vi "DisplayJson.vi"(11 "JSON String In":string="[{\"version\":\"1.0.0\",\"header\":{\"creationDate\":\"2022-06-03T00:00:00\",\"remarks\":\"\",\"serialNumber\":\"98172\",\"productNumber\":\"123021.1804\",\"productType\":\"PAA-9L\",\"pressureType\":2,\"productSeries\":\"9L\",\"compensatedTemperatureRange\":{\"min\":-10.0,\"max\":80.0,\"unit\":4},\"compensatedPressureRange\":{\"min\":0.0,\"max\":0.35,\"unit\":3},\"electricSupply\":{\"magnitude\":1.0,\"unit\":18},\"orderNumber\":9990266,\"orderPosition\":3,\"orderTargetDispatchDate\":\"2022-06-02T00:00:00+00:00\",\"customerName\":\"DemoData Inc.\",\"customerNumber\":12345678,\"customerOrderNumber\":\"Cust-9990266-123\",\"customerReferenceNumber\":\"\",\"customerProductT...") -> ()   [LabVIEW 2017] (continued)
\"temperature\":{\"output\":{\"magnitude\":19.5449,\"unit\":4},\"error\":{\"magnitude\":-0.0059422599,\"unit\":4}}}}}},{\"reference\":\"F_12300_XX_0000098765\",\"environmentTarget\":{\"pressure\":{\"magnitude\":0.11,\"unit\":3},\"temperature\":{\"magnitude\":20.0,\"unit\":4}},\"environment\":{\"pressure\":{\"magnitude\":0.11,\"unit\":3},\"temperature\":{\"magnitude\":19.5509,\"unit\":4},\"supply\":{\"magnitude\":1.0,\"unit\":18}},\"raw\":{\"signal\":{\"magnitude\":26.416661534,\"unit\":22},\"bridgeResistance\":{\"magnitude\":3495.5999199,\"unit\":28}},\"compensated\":{\"mathematicalModels\":{\"MM0123\":{\"pressure\":{\"output\":{\"magnitude\":0.109977,\"unit\":3},\"error\":{\"magnitude\":-0.0065360975,\"unit\":7}},\"temperature\":{\"output\":{\"magnitude\":19.5426,\"unit\":4},\"error\":{\"magnitude\":-0.0082689775,\"unit\":4}}}}}},{\"reference\":\"F_12300_XX_0000098765\",\"environmentTarget\":{\"pressure\":{\"magnitude\":0.19,\"unit\":3},\"temperature\":{\"magnitude\":20.0,\"unit\":4}},\"environment\":{\"pressure\":{\"magnitude\":0.189998,\"unit\":3},\"temperature\":{\"magnitude\":19.5509,\"unit\":4},\"supply\":{\"magnitude\":1.0,\"unit\":18}},\"raw\":{\"signal\":{\"magnitude\":37.030268769,\"unit\":22},\"bridgeResistance\":{\"magnitude\":3491.6224563,\"unit\":28}},\"compensated\":{\"mathematicalModels\":{\"MM0123\":{\"pressure\":{\"output\":{\"magnitude\":0.190007,\"unit\":3},\"error\":{\"magnitude\":0.0024560994,\"unit\":7}},\"temperature\":{\"output\":{\"magnitude\":19.5389,\"unit\":4},\"error\":{\"magnitude\":-0.012049357,\"unit\":4}}}}}},{\"reference\":\"F_12300_XX_0000098765\",\"environmentTarget\":{\"pressure\":{\"magnitude\":0.27,\"unit\":3},\"temperature\":{\"magnitude\":20.0,\"unit\":4}},\"environment\":{\"pressure\":{\"magnitude\":0.269994,\"unit\":3},\"temperature\":{\"magnitude\":19.5509,\"unit\":4},\"supply\":{\"magnitude\":1.0,\"unit\":18}},\"raw\":{\"signal\":{\"magnitude\":47.60635601,\"unit\":22},\"bridgeResistance\":{\"magnitude\":3487.7228678,\"unit\":28}},\"compensated\":{\"mathematicalModels\":{\"MM0123\":{\"pressure\":{\"output\":{\"magnitude\":0.270015,\"unit\":3},\"error\":{\"magnitude\":0.0061300393,\"unit\":7}},\"temperature\":{\"output\":{\"magnitude\":19.5358,\"unit\":4},\"error\":{\"magnitude\":-0.015037284,\"unit\":4}}}}}},{\"reference\":\"F_12300_XX_0000098765\",\"environmentTarget\":{\"pressure\":{\"magnitude\":0.35,\"unit\":3},\"temperature\":{\"magnitude\":20.0,\"unit\":4}},\"environment\":{\"pressure\":{\"magnitude\":0.35,\"unit\":3},\"temperature\":{\"magnitude\":19.5509,\"unit\":4},\"supply\":{\"magnitude\":1.0,\"unit\":18}},\"raw\":{\"signal\":{\"magnitude\":58.14484892,\"unit\":22},\"bridgeResistance\":{\"magnitude\":3483.890155,\"unit\":28}},\"compensated\":{\"mathematicalModels\":{\"MM0123\":{\"pressure\":{\"output\":{\"magnitude\":0.350003,\"unit\":3},\"error\":{\"magnitude\":0.00098441802,\"unit\":7}},\"temperature\":{\"output\":{\"magnitude\":19.5323,\"unit\":4},\"error\":{\"magnitude\":-0.018584481,\"unit\":4}}}}}},{\"reference\":\"F_12300_XX_0000098765\",\"environmentTarget\":{\"pressure\":{\"magnitude\":0.03,\"unit\":3},\"temperature\":{\"magnitude\":40.0,\"unit\":4}},\"environment\":{\"pressure\":{\"magnitude\":0.0300037,\"unit\":3},\"temperature\":{\"magnitude\":39.7284,\"unit\":4},\"supply\":{\"magnitude\":1.0,\"unit\":18}},\"raw\":{\"signal\":{\"magnitude\":16.748092375,\"unit\":22},\"bridgeResistance\":{\"magnitude\":3674.5848343,\"unit\":28}},\"compensated\":{\"mathematicalModels\":{\"MM0123\":{\"pressure\":{\"output\":{\"magnitude\":0.0300189,\"unit\":3},\"error\":{\"magnitude\":0.004330657,\"unit\":7}},\"temperature\":{\"output\":{\"magnitude\":39.7229,\"unit\":4},\"error\":{\"magnitude\":-0.005475721,\"unit\":4}}}}}},{\"reference\":\"F_12300_XX_0000098765\",\"environmentTarget\":{\"pressure\":{\"magnitude\":0.11,\"unit\":3},\"temperature\":{\"magnitude\":40.0,\"unit\":4}},\"environment\":{\"pressure\":{\"magnitude\":0.110002,\"unit\":3},\"temperature\":{\"magnitude\":39.7284,\"unit\":4},\"supply\":{\"magnitude\":1.0,\"unit\":18}},\"raw\":{\"signal\":{\"magnitude\":27.434150149,\"unit\":22},\"bridgeResistance\":{\"magnitude\":3670.5212952,\"unit\":28}},\"compensated\":{\"mathematicalModels\":{\"MM0123\":{\"pressure\":{\"output\":{\"magnitude\":0.109982,\"unit\":3},\"error\":{\"magnitude\":-0.0057516302,\"unit\":7}},\"temperature\":{\"output\":{\"magnitude\":39.7229,\"unit\":4},\"error\":{\"magnitude\":-0.0055694235,\"unit\":4}}}}}},{\"reference\":\"F_12300_XX_0000098765\",\"environmentTarget\":{\"pressure\":{\"magnitude\":0.19,\"unit\":3},\"temperature\":{\"magnitude\":40.0,\"unit\":4}},\"environment\":{\"pressure\":{\"magnitude\":0.190005,\"unit\":3},\"temperature\":{\"magnitude\":39.7284,\"unit\":4},\"supply\":{\"magnitude\":1.0,\"unit\":18}},\"raw\":{\"signal\":{\"magnitude\":38.097016772,\"unit\":22},\"bridgeResistance\":{\"magnitude\":3666.4814116,\"unit\":28}},\"compensated\":{\"mathematicalModels\":{\"MM0123\":{\"pressure\":{\"output\":{\"magnitude\":0.190006,\"unit\":3},\"error\":{\"magnitude\":0.0004046361,\"unit\":7}},\"temperature\":{\"output\":{\"magnitude\":39.7178,\"unit\":4},\"error\":{\"magnitude\":-0.010669287,\"unit\":4}}}}}},{\"reference\":\"F_12300_XX_0000098765\",\"environmentTarget\":{\"pressure\":{\"magnitude\":0.27,\"unit\":3},\"temperature\":{\"magnitude\":40.0,\"unit\":4}},\"environment\":{\"pressure\":{\"magnitude\":0.269997,\"unit\":3},\"temperature\":{\"magnitude\":39.7284,\"unit\":4},\"supply\":{\"magnitude\":1.0,\"unit\":18}},\"raw\":{\"signal\":{\"magnitude\":48.726177501,\"unit\":22},\"bridgeResistance\":{\"magnitude\":3662.5874392,\"unit\":28}},\"compensated\":{\"mathematicalModels\":{\"MM0123\":{\"pressure\":{\"output\":{\"magnitude\":0.270008,\"unit\":3},\"error\":{\"magnitude\":0.0031543513,\"unit\":7}},\"temperature\":{\"output\":{\"magnitude\":39.7206,\"unit\":4},\"error\":{\"magnitude\":-0.0078327671,\"unit\":4}}}}}},{\"reference\":\"F_12300_XX_0000098765\",\"environmentTarget\":{\"pressure\":{\"magnitude\":0.35,\"unit\":3},\"temperature\":{\"magnitude\":40.0,\"unit\":4}},\"environment\":{\"pressure\":{\"magnitude\":0.350003,\"unit\":3},\"temperature\":{\"magnitude\":39.7284,\"unit\":4},\"supply\":{\"magnitude\":1.0,\"unit\":18}},\"raw\":{\"signal\":{\"magnitude\":59.320792825,\"unit\":22},\"bridgeResistance\":{\"magnitude\":3658.7134123,\"unit\":28}},\"compensated\":{\"mathematicalModels\":{\"MM0123\":{\"pressure\":{\"output\":{\"magnitude\":0.349986,\"unit\":3},\"error\":{\"magnitude\":-0.0048622518,\"unit\":7}},\"temperature\":{\"output\":{\"magnitude\":39.7176,\"unit\":4},\"error\":{\"magnitude\":-0.010854606,\"unit\":4}}}}}},{\"reference\":\"F_12300_XX_0000098765\",\"environmentTarget\":{\"pressure\":{\"magnitude\":0.03,\"unit\":3},\"temperature\":{\"magnitude\":60.0,\"unit\":4}},\"environment\":{\"pressure\":{\"magnitude\":0.0299911,\"unit\":3},\"temperature\":{\"magnitude\":59.8651,\"unit\":4},\"supply\":{\"magnitude\":1.0,\"unit\":18}},\"raw\":{\"signal\":{\"magnitude\":17.813294413,\"unit\":22},\"bridgeResistance\":{\"magnitude\":3866.6561439,\"unit\":28}},\"compensated\":{\"mathematicalModels\":{\"MM0123\":{\"pressure\":{\"output\":{\"magnitude\":0.0299973,\"unit\":3},\"error\":{\"magnitude\":0.0017700015,\"unit\":7}},\"temperature\":{\"output\":{\"magnitude\":59.9259,\"unit\":4},\"error\":{\"magnitude\":0.06081023,\"unit\":4}}}}}},{\"reference\":\"F_12300_XX_0000098765\",\"environmentTarget\":{\"pressure\":{\"magnitude\":0.11,\"unit\":3},\"temperature\":{\"magnitude\":60.0,\"unit\":4}},\"environment\":{\"pressure\":{\"magnitude\":0.109995,\"unit\":3},\"temperature\":{\"magnitude\":59.8651,\"unit\":4},\"supply\":{\"magnitude\":1.0,\"unit\":18}},\"raw\":{\"signal\":{\"magnitude\":28.584875218,\"unit\":22},\"bridgeResistance\":{\"magnitude\":3862.5400232,\"unit\":28}},\"compensated\":{\"mathematicalModels\":{\"MM0123\":{\"pressure\":{\"output\":{\"magnitude\":0.109979,\"unit\":3},\"error\":{\"magnitude\":-0.0046951087,\"unit\":7}},\"temperature\":{\"output\":{\"magnitude\":59.9272,\"unit\":4},\"error\":{\"magnitude\":0.062078048,\"unit\":4}}}}}},{\"reference\":\"F_12300_XX_0000098765\",\"environmentTarget\":{\"pressure\":{\"magnitude\":0.19,\"unit\":3},\"temperature\":{\"magnitude\":60.0,\"unit\":4}},\"environment\":{\"pressure\":{\"magnitude\":0.190004,\"unit\":3},\"temperature\":{\"magnitude\":59.8651,\"unit\":4},\"supply\":{\"magnitude\":1.0,\"unit\":18}},\"raw\":{\"signal\":{\"magnitude\":39.33493725,\"unit\":22},\"bridgeResistance\":{\"magnitude\":3858.4848982,\"unit\":28}},\"compensated\":{\"mathematicalModels\":{\"MM0123\":{\"pressure\":{\"output\":{\"magnitude\":0.190003,\"unit\":3},\"error\":{\"magnitude\":-0.00025005669,\"unit\":7}},\"temperature\":{\"output\":{\"magnitude\":59.9287,\"unit\":4},\"error\":{\"magnitude\":0.063577803,\"unit\":4}}}}}},{\"reference\":\"F_12300_XX_0000098765\",\"environmentTarget\":{\"pressure\":{\"magnitude\":0.27,\"unit\":3},\"temperature\":{\"magnitude\":60.0,\"unit\":4}},\"environment\":{\"pressure\":{\"magnitude\":0.270004,\"unit\":3},\"temperature\":{\"magnitude\":59.8651,\"unit\":4},\"supply\":{\"magnitude\":1.0,\"unit\":18}},\"raw\":{\"signal\":{\"magnitude\":50.057189453,\"unit\":22},\"bridgeResistance\":{\"magnitude\":3854.4965821,\"unit\":28}},\"compensated\":{\"mathematicalModels\":{\"MM0123\":{\"pressure\":{\"output\":{\"magnitude\":0.270024,\"unit\":3},\"error\":{\"magnitude\":0.0057789716,\"unit\":7}},\"temperature\":{\"output\":{\"magnitude\":59.9307,\"unit\":4},\"error\":{\"magnitude\":0.065552658,\"unit\":4}}}}}},{\"reference\":\"F_12300_XX_0000098765\",\"environmentTarget\":{\"pressure\":{\"magnitude\":0.35,\"unit\":3},\"temperature\":{\"magnitude\":60.0,\"unit\":4}},\"environment\":{\"pressure\":{\"magnitude\":0.349995,\"unit\":3},\"temperature\":{\"magnitude\":59.8651,\"unit\":4},\"supply\":{\"magnitude\":1.0,\"unit\":18}},\"raw\":{\"signal\":{\"magnitude\":60.744545032,\"unit\":22},\"bridgeResistance\":{\"magnitude\":3850.5667489,\"unit\":28}},\"compensated\":{\"mathematicalModels\":{\"MM0123\":{\"pressure\":{\"output\":{\"magnitude\":0.349989,\"unit\":3},\"error\":{\"magnitude\":-0.0016070127,\"unit\":7}},\"temperature\":{\"output\":{\"magnitude\":59.9319,\"unit\":4},\"error\":{\"magnitude\":0.06679753,\"unit\":4}}}}}},{\"reference\":\"F_12300_XX_0000098765\",\"environmentTarget\":{\"pressure\":{\"magnitude\":0.03,\"unit\":3},\"temperature\":{\"magnitude\":80.0,\"unit\":4}},\"environment\":{\"pressure\":{\"magnitude\":0.0300046,\"unit\":3},\"temperature\":{\"magnitude\":79.9513,\"unit\":4},\"supply\":{\"magnitude\":1.0,\"unit\":18}},\"raw\":{\"signal\":{\"magnitude\":19.002144905,\"unit\":22},\"bridgeResistance\":{\"magnitude\":4072.8231737,\"unit\":28}},\"compensated\":{\"mathematicalModels\":{\"MM0123\":{\"pressure\":{\"output\":{\"magnitude\":0.0300206,\"unit\":3},\"error\":{\"magnitude\":0.004584639,\"unit\":7}},\"temperature\":{\"output\":{\"magnitude\":80.0436,\"unit\":4},\"error\":{\"magnitude\":0.092214141,\"unit\":4}}}}}},{\"reference\":\"F_12300_XX_0000098765\",\"environmentTarget\":{\"pressure\":{\"magnitude\":0.11,\"unit\":3},\"temperature\":{\"magnitude\":80.0,\"unit\":4}},\"environment\":{\"pressure\":{\"magnitude\":0.110002,\"unit\":3},\"temperature\":{\"magnitude\":79.9513,\"unit\":4},\"supply\":{\"magnitude\":1.0,\"unit\":18}},\"raw\":{\"signal\":{\"magnitude\":29.879764386,\"unit\":22},\"bridgeResistance\":{\"magnitude\":4068.6482783,\"unit\":28}},\"compensated\":{\"mathematicalModels\":{\"MM0123\":{\"pressure\":{\"output\":{\"magnitude\":0.109968,\"unit\":3},\"error\":{\"magnitude\":-0.0096781592,\"unit\":7}},\"temperature\":{\"output\":{\"magnitude\":80.0462,\"unit\":4},\"error\":{\"magnitude\":0.094857113,\"unit\":4}}}}}},{\"reference\":\"F_12300_XX_0000098765\",\"environmentTarget\":{\"pressure\":{\"magnitude\":0.19,\"unit\":3},\"temperature\":{\"magnitude\":80.0,\"unit\":4}},\"environment\":{\"pressure\":{\"magnitude\":0.189994,\"unit\":3},\"temperature\":{\"magnitude\":79.9513,\"unit\":4},\"supply\":{\"magnitude\":1.0,\"unit\":18}},\"raw\":{\"signal\":{\"magnitude\":40.746012852,\"unit\":22},\"bridgeResistance\":{\"magnitude\":4064.5654978,\"unit\":28}},\"compensated\":{\"mathematicalModels\":{\"MM0123\":{\"pressure\":{\"output\":{\"magnitude\":0.190002,\"unit\":3},\"error\":{\"magnitude\":0.0022412163,\"unit\":7}},\"temperature\":{\"output\":{\"magnitude\":80.0536,\"unit\":4},\"error\":{\"magnitude\":0.1022268,\"unit\":4}}}}}},{\"reference\":\"F_12300_XX_0000098765\",\"environmentTarget\":{\"pressure\":{\"magnitude\":0.27,\"unit\":3},\"temperature\":{\"magnitude\":80.0,\"unit\":4}},\"environment\":{\"pressure\":{\"magnitude\":0.270005,\"unit\":3},\"temperature\":{\"magnitude\":79.9513,\"unit\":4},\"supply\":{\"magnitude\":1.0,\"unit\":18}},\"raw\":{\"signal\":{\"magnitude\":51.587537274,\"unit\":22},\"bridgeResistance\":{\"magnitude\":4060.5136813,\"unit\":28}},\"compensated\":{\"mathematicalModels\":{\"MM0123\":{\"pressure\":{\"output\":{\"magnitude\":0.270027,\"unit\":3},\"error\":{\"magnitude\":0.0064070438,\"unit\":7}},\"temperature\":{\"output\":{\"magnitude\":80.0595,\"unit\":4},\"error\":{\"magnitude\":0.10820001,\"unit\":4}}}}}},{\"reference\":\"F_12300_XX_0000098765\",\"environmentTarget\":{\"pressure\":{\"magnitude\":0.35,\"unit\":3},\"temperature\":{\"magnitude\":80.0,\"unit\":4}},\"environment\":{\"pressure\":{\"magnitude\":0.349997,\"unit\":3},\"temperature\":{\"magnitude\":79.9513,\"unit\":4},\"supply\":{\"magnitude\":1.0,\"unit\":18}},\"raw\":{\"signal\":{\"magnitude\":62.396098066,\"unit\":22},\"bridgeResistance\":{\"magnitude\":4056.4915818,\"unit\":28}},\"compensated\":{\"mathematicalModels\":{\"MM0123\":{\"pressure\":{\"output\":{\"magnitude\":0.349985,\"unit\":3},\"error\":{\"magnitude\":-0.0034619433,\"unit\":7}},\"temperature\":{\"output\":{\"magnitude\":80.0638,\"unit\":4},\"error\":{\"magnitude\":0.11240626,\"unit\":4}}}}}}]},{\"version\":\"1.0.0\",\"header\":{\"creationDate\":\"2022-06-03T00:00:00\",\"remarks\":\"\",\"serialNumber\":\"98083\",\"productNumber\":\"123021.1804\",\"productType\":\"PAA-9L\",\"pressureType\":2,\"productSeries\":\"9L\",\"compensatedTemperatureRange\":{\"min\":-10.0,\"max\":80.0,\"unit\":4},\"compensatedPressureRange\":{\"min\":0.0,\"max\":0.35,\"unit\":3},\"electricSupply\":{\"magnitude\":1.0,\"unit\":18},\"orderNumber\":9990266,\"orderPosition\":3,\"orderTargetDispatchDate\":\"2022-06-02T00:00:00+00:00\",\"customerName\":\"DemoData Inc.\",\"customerNumber\":12345678,\"customerOrderNumber\":\"Cust-9990266-123\",\"customerReferenceNumber\":\"\",\"customerProductType\":\"123021-1804 Rev.AA\"},\"compensationMethods\":{\"mathematicalModels\":{\"MM0123\":{\"modelType\":\"MM0123\",\"productNumber\":\"000000.0000\",\"compensatedTemperatureRange\":{\"min\":-10.0,\"max\":80.0,\"unit\":4},\"compensatedPressureRange\":{\"min\":0.0,\"max\":0.35,\"unit\":3},\"electricSupply\":{\"magnitude\":1.0,\"unit\":18},\"parts\":{\"pressure\":{\"inputs\":[\"Sig\",\"R\"],\"output\":\"P\",\"description\":\"P = f(Sig,R)\",\"coefficients\":[[3.63310435718,-0.00363389206026,1.34930392587E-06,-2.24563835828E-10,1.39905821744E-14],[-0.0993877484134,0.000105975761375,-3.95803321041E-08,6.56139178036E-12,-4.08510736386E-16],[-0.000366248546746,4.19017408478E-07,-1.77205627573E-10,3.30128020446E-14,-2.29210272903E-18]]},\"temperature\":{\"inputs\":[\"R\",\"Sig\"],\"output\":\"T\",\"description\":\"T = f(R,Sig)\",\"coefficients\":[[-7824.08516559,-7.6450274546,0.0655428608171],[7.6820085907,0.00943972080923,-7.29339544197E-05],[-0.0028951031634,-4.23164182833E-06,3.02382272713E-08],[4.94544252506E-07,8.27138238584E-10,-5.54321442715E-12],[-3.18956234296E-11,-5.97910707007E-14,3.79410156991E-16]]}}}}},\"measurements\":[{\"reference\":\"F_12300_XX_0000098765\",\"environmentTarget\":{\"pressure\":{\"magnitude\":0.03,\"unit\":3},\"temperature\":{\"magnitude\":-10.0,\"unit\":4}},\"environment\":{\"pressure\":{\"magnitude\":0.029998,\"unit\":3},\"temperature\":{\"magnitude\":-10.7286,\"unit\":4},\"supply\":{\"magnitude\":1.0,\"unit\":18}},\"raw\":{\"signal\":{\"magnitude\":15.768740367,\"unit\":22},\"bridgeResistance\":{\"magnitude\":3289.7518235,\"unit\":28}},\"compensated\":{\"mathematicalModels\":{\"MM0123\":{\"pressure\":{\"output\":{\"magnitude\":0.0300118,\"unit\":3},\"error\":{\"magnitude\":0.0039552178,\"unit\":7}},\"temperature\":{\"output\":{\"magnitude\":-10.8423,\"unit\":4},\"error\":{\"magnitude\":-0.11370704,\"unit\":4}}}}}},{\"reference\":\"F_12300_XX_0000098765\",\"environmentTarget\":{\"pressure\":{\"magnitude\":0.11,\"unit\":3},\"temperature\":{\"magnitude\":-10.0,\"unit\":4}},\"environment\":{\"pressure\":{\"magnitude\":0.110009,\"unit\":3},\"temperature\":{\"magnitude\":-10.7286,\"unit\":4},\"supply\":{\"magnitude\":1.0,\"unit\":18}},\"raw\":{\"signal\":{\"magnitude\":27.663432001,\"unit\":22},\"bridgeResistance\":{\"magnitude\":3284.2425899,\"unit\":28}},\"compensated\":{\"mathematicalModels\":{\"MM0123\":{\"pressure\":{\"output\":{\"magnitude\":0.109973,\"unit\":3},\"error\":{\"magnitude\":-0.010313162,\"unit\":7}},\"temperature\":{\"output\":{\"magnitude\":-10.8468,\"unit\":4},\"error\":{\"magnitude\":-0.1181895,\"unit\":4}}}}}},{\"reference\":\"F_12300_XX_0000098765\",\"environmentTarget\":{\"pressure\":{\"magnitude\":0.19,\"unit\":3},\"temperature\":{\"magnitude\":-10.0,\"unit\":4}},\"environment\":{\"pressure\":{\"magnitude\":0.190006,\"unit\":3},\"temperature\":{\"magnitude\":-10.7286,\"unit\":4},\"supply\":{\"magnitude\":1.0,\"unit\":18}},\"raw\":{\"signal\":{\"magnitude\":39.521415848,\"unit\":22},\"bridgeResistance\":{\"magnitude\":3279.8976313,\"unit\":28}},\"compensated\":{\"mathematicalModels\":{\"MM0123\":{\"pressure\":{\"output\":{\"magnitude\":0.190016,\"unit\":3},\"error\":{\"magnitude\":0.0029939943,\"unit\":7}},\"temperature\":{\"output\":{\"magnitude\":-10.8438,\"unit\":4},\"error\":{\"magnitude\":-0.11516709,\"unit\":4}}}}}},{\"reference\":\"F_12300_XX_0000098765\",\"environmentTarget\":{\"pressure\":{\"magnitude\":0.27,\"unit\":3},\"temperature\":{\"magnitude\":-10.0,\"unit\":4}},\"environment\":{\"pressure\":{\"magnitude\":0.270006,\"unit\":3},\"temperature\":{\"magnitude\":-10.7286,\"unit\":4},\"supply\":{\"magnitude\":1.0,\"unit\":18}},\"raw\":{\"signal\":{\"magnitude\":51.326682167,\"unit\":22},\"bridgeResistance\":{\"magnitude\":3275.6600996,\"unit\":28}},\"compensated\":{\"mathematicalModels\":{\"MM0123\":{\"pressure\":{\"output\":{\"magnitude\":0.270037,\"unit\":3},\"error\":{\"magnitude\":0.0089972975,\"unit\":7}},\"temperature\":{\"output\":{\"magnitude\":-10.8382,\"unit\":4},\"error\":{\"magnitude\":-0.10956906,\"unit\":4}}}}}},{\"reference\":\"F_12300_XX_0000098765\",\"environmentTarget\":{\"pressure\":{\"magnitude\":0.35,\"unit\":3},\"temperature\":{\"magnitude\":-10.0,\"unit\":4}},\"environment\":{\"pressure\":{\"magnitude\":0.35,\"unit\":3},\"temperature\":{\"magnitude\":-10.7286,\"unit\":4},\"supply\":{\"magnitude\":1.0,\"unit\":18}},\"raw\":{\"signal\":{\"magnitude\":63.072780161,\"unit\":22},\"bridgeResistance\":{\"magnitude\":3271.4490528,\"unit\":28}},\"compensated\":{\"mathematicalModels\":{\"MM0123\":{\"pressure\":{\"output\":{\"magnitude\":0.349995,\"unit\":3},\"error\":{\"magnitude\":-0.0014930458,\"unit\":7}},\"temperature\":{\"output\":{\"magnitude\":-10.8469,\"unit\":4},\"error\":{\"magnitude\":-0.11824585,\"unit\":4}}}}}},{\"reference\":\"F_12300_XX_0000098765\",\"environmentTarget\":{\"pressure\":{\"magnitude\":0.03,\"unit\":3},\"temperature\":{\"magnitude\":0.0,\"unit\":4}},\"environment\":{\"pressure\":{\"magnitude\":0.0299993,\"unit\":3},\"temperature\":{\"magnitude\":-0.629962,\"unit\":4},\"supply\":{\"magnitude\":1.0,\"unit\":18}},\"raw\":{\"signal\":{\"magnitude\":16.265941035,\"unit\":22},\"bridgeResistance\":{\"magnitude\":3359.1605663,\"unit\":28}},\"compensated\":{\"mathematicalModels\":{\"MM0123\":{\"pressure\":{\"output\":{\"magnitude\":0.0300172,\"unit\":3},\"error\":{\"magnitude\":0.0051262489,\"unit\":7}},\"temperature\":{\"output\":{\"magnitude\":-0.751572,\"unit\":4},\"error\":{\"magnitude\":-0.1216099,\"unit\":4}}}}}},{\"reference\":\"F_12300_XX_0000098765\",\"environmentTarget\":{\"pressure\":{\"magnitude\":0.11,\"unit\":3},\"temperature\":{\"magnitude\":0.0,\"unit\":4}},\"environment\":{\"pressure\":{\"magnitude\":0.110001,\"unit\":3},\"temperature\":{\"magnitude\":-0.629962,\"unit\":4},\"supply\":{\"magnitude\":1.0,\"unit\":18}},\"raw\":{\"signal\":{\"magnitude\":28.125684179,\"unit\":22},\"bridgeResistance\":{\"magnitude\":3354.6447949,\"unit\":28}},\"compensated\":{\"mathematicalModels\":{\"MM0123\":{\"pressure\":{\"output\":{\"magnitude\":0.109972,\"unit\":3},\"error\":{\"magnitude\":-0.0083468924,\"unit\":7}},\"temperature\":{\"output\":{\"magnitude\":-0.756891,\"unit\":4},\"error\":{\"magnitude\":-0.12692921,\"unit\":4}}}}}},{\"reference\":\"F_12300_XX_0000098765\",\"environmentTarget\":{\"pressure\":{\"magnitude\":0.19,\"unit\":3},\"temperature\":{\"magnitude\":0.0,\"unit\":4}},\"environment\":{\"pressure\":{\"magnitude\":0.190006,\"unit\":3},\"temperature\":{\"magnitude\":-0.629962,\"unit\":4},\"supply\":{\"magnitude\":1.0,\"unit\":18}},\"raw\":{\"signal\":{\"magnitude\":39.949259633,\"unit\":22},\"bridgeResistance\":{\"magnitude\":3350.2650804,\"unit\":28}},\"compensated\":{\"mathematicalModels\":{\"MM0123\":{\"pressure\":{\"output\":{\"magnitude\":0.19,\"unit\":3},\"error\":{\"magnitude\":-0.001845037,\"unit\":7}},\"temperature\":{\"output\":{\"magnitude\":-0.757234,\"unit\":4},\"error\":{\"magnitude\":-0.12727247,\"unit\":4}}}}}},{\"reference\":\"F_12300_XX_0000098765\",\"environmentTarget\":{\"pressure\":{\"magnitude\":0.27,\"unit\":3},\"temperature\":{\"magnitude\":0.0,\"unit\":4}},\"environment\":{\"pressure\":{\"magnitude\":0.269995,\"unit\":3},\"temperature\":{\"magnitude\":-0.629962,\"unit\":4},\"supply\":{\"magnitude\":1.0,\"unit\":18}},\"raw\":{\"signal\":{\"magnitude\":51.72348672,\"unit\":22},\"bridgeResistance\":{\"magnitude\":3345.9485402,\"unit\":28}},\"compensated\":{\"mathematicalModels\":{\"MM0123\":{\"pressure\":{\"output\":{\"magnitude\":0.270016,\"unit\":3},\"error\":{\"magnitude\":0.0058723742,\"unit\":7}},\"temperature\":{\"output\":{\"magnitude\":-0.763469,\"unit\":4},\"error\":{\"magnitude\":-0.1335069,\"unit\":4}}}}}},{\"reference\":\"F_12300_XX_0000098765\",\"environmentTarget\":{\"pressure\":{\"magnitude\":0.35,\"unit\":3},\"temperature\":{\"magnitude\":0.0,\"unit\":4}},\"environment\":{\"pressure\":{\"magnitude\":0.350003,\"unit\":3},\"temperature\":{\"magnitude\":-0.629962,\"unit\":4},\"supply\":{\"magnitude\":1.0,\"unit\":18}},\"raw\":{\"signal\":{\"magnitude\":63.441446846,\"unit\":22},\"bridgeResistance\":{\"magnitude\":3341.7747282,\"unit\":28}},\"compensated\":{\"mathematicalModels\":{\"MM0123\":{\"pressure\":{\"output\":{\"magnitude\":0.34997,\"unit\":3},\"error\":{\"magnitude\":-0.009570085,\"unit\":7}},\"temperature\":{\"output\":{\"magnitude\":-0.765087,\"unit\":4},\"error\":{\"magnitude\":-0.1351251,\"unit\":4}}}}}},{\"reference\":\"F_12300_XX_0000098765\",\"environmentTarget\":{\"pressure\":{\"magnitude\":0.03,\"unit\":3},\"temperature\":{\"magnitude\":20.0,\"unit\":4}},\"environment\":{\"pressure\":{\"magnitude\":0.0299954,\"unit\":3},\"temperature\":{\"magnitude\":19.5509,\"unit\":4},\"supply\":{\"magnitude\":1.0,\"unit\":18}},\"raw\":{\"signal\":{\"magnitude\":17.297816417,\"unit\":22},\"bridgeResistance\":{\"magnitude\":3516.9951878,\"unit\":28}},\"compensated\":{\"mathematicalModels\":{\"MM0123\":{\"pressure\":{\"output\":{\"magnitude\":0.0300062,\"unit\":3},\"error\":{\"magnitude\":0.0030915574,\"unit\":7}},\"temperature\":{\"output\":{\"magnitude\":19.5472,\"unit\":4},\"error\":{\"magnitude\":-0.0036683152,\"unit\":4}}}}}},{\"reference\":\"F_12300_XX_0000098765\",\"environmentTarget\":{\"pressure\":{\"magnitude\":0.11,\"unit\":3},\"temperature\":{\"magnitude\":20.0,\"unit\":4}},\"environment\":{\"pressure\":{\"magnitude\":0.109995,\"unit\":3},\"temperature\":{\"magnitude\":19.5509,\"unit\":4},\"supply\":{\"magnitude\":1.0,\"unit\":18}},\"raw\":{\"signal\":{\"magnitude\":29.147457751,\"unit\":22},\"bridgeResistance\":{\"magnitude\":3512.4984667,\"unit\":28}},\"compensated\":{\"mathematicalModels\":{\"MM0123\":{\"pressure\":{\"output\":{\"magnitude\":0.109965,\"unit\":3},\"error\":{\"magnitude\":-0.0084408516,\"unit\":7}},\"temperature\":{\"output\":{\"magnitude\":19.543,\"unit\":4},\"error\":{\"magnitude\":-0.0078639068,\"unit\":4}}}}}},{\"reference\":\"F_12300_XX_0000098765\",\"environmentTarget\":{\"pressure\":{\"magnitude\":0.19,\"unit\":3},\"temperature\":{\"magnitude\":20.0,\"unit\":4}},\"environment\":{\"pressure\":{\"magnitude\":0.190002,\"unit\":3},\"temperature\":{\"magnitude\":19.5509,\"unit\":4},\"supply\":{\"magnitude\":1.0,\"unit\":18}},\"raw\":{\"signal\":{\"magnitude\":40.967596289,\"unit\":22},\"bridgeResistance\":{\"magnitude\":3508.1412376,\"unit\":28}},\"compensated\":{\"mathematicalModels\":{\"MM0123\":{\"pressure\":{\"output\":{\"magnitude\":0.190009,\"unit\":3},\"error\":{\"magnitude\":0.0019583559,\"unit\":7}},\"temperature\":{\"output\":{\"magnitude\":19.5457,\"unit\":4},\"error\":{\"magnitude\":-0.0051906945,\"unit\":4}}}}}},{\"reference\":\"F_12300_XX_0000098765\",\"environmentTarget\":{\"pressure\":{\"magnitude\":0.27,\"unit\":3},\"temperature\":{\"magnitude\":20.0,\"unit\":4}},\"environment\":{\"pressure\":{\"magnitude\":0.26999,\"unit\":3},\"temperature\":{\"magnitude\":19.5509,\"unit\":4},\"supply\":{\"magnitude\":1.0,\"unit\":18}},\"raw\":{\"signal\":{\"magnitude\":52.741361922,\"unit\":22},\"bridgeResistance\":{\"magnitude\":3503.7893624,\"unit\":28}},\"compensated\":{\"mathematicalModels\":{\"MM0123\":{\"pressure\":{\"output\":{\"magnitude\":0.270029,\"unit\":3},\"error\":{\"magnitude\":0.011218428,\"unit\":7}},\"temperature\":{\"output\":{\"magnitude\":19.538,\"unit\":4},\"error\":{\"magnitude\":-0.012843363,\"unit\":4}}}}}},{\"reference\":\"F_12300_XX_0000098765\",\"environmentTarget\":{\"pressure\":{\"magnitude\":0.35,\"unit\":3},\"temperature\":{\"magnitude\":20.0,\"unit\":4}},\"environment\":{\"pressure\":{\"magnitude\":0.350004,\"unit\":3},\"temperature\":{\"magnitude\":19.5509,\"unit\":4},\"supply\":{\"magnitude\":1.0,\"unit\":18}},\"raw\":{\"signal\":{\"magnitude\":64.467097155,\"unit\":22},\"bridgeResistance\":{\"magnitude\":3499.5857801,\"unit\":28}},\"compensated\":{\"mathematicalModels\":{\"MM0123\":{\"pressure\":{\"output\":{\"magnitude\":0.350009,\"unit\":3},\"error\":{\"magnitude\":0.0013639933,\"unit\":7}},\"temperature\":{\"output\":{\"magnitude\":19.5374,\"unit\":4},\"error\":{\"magnitude\":-0.013502905,\"unit\":4}}}}}},{\"reference\":\"F_12300_XX_0000098765\",\"environmentTarget\":{\"pressure\":{\"magnitude\":0.03,\"unit\":3},\"temperature\":{\"magnitude\":40.0,\"unit\":4}},\"environment\":{\"pressure\":{\"magnitude\":0.0299955,\"unit\":3},\"temperature\":{\"magnitude\":39.7284,\"unit\":4},\"supply\":{\"magnitude\":1.0,\"unit\":18}},\"raw\":{\"signal\":{\"magnitude\":18.397808565,\"unit\":22},\"bridgeResistance\":{\"magnitude\":3693.5579638,\"unit\":28}},\"compensated\":{\"mathematicalModels\":{\"MM0123\":{\"pressure\":{\"output\":{\"magnitude\":0.0300132,\"unit\":3},\"error\":{\"magnitude\":0.0050623537,\"unit\":7}},\"temperature\":{\"output\":{\"magnitude\":39.7198,\"unit\":4},\"error\":{\"magnitude\":-0.0086558786,\"unit\":4}}}}}},{\"reference\":\"F_12300_XX_0000098765\",\"environmentTarget\":{\"pressure\":{\"magnitude\":0.11,\"unit\":3},\"temperature\":{\"magnitude\":40.0,\"unit\":4}},\"environment\":{\"pressure\":{\"magnitude\":0.109995,\"unit\":3},\"temperature\":{\"magnitude\":39.7284,\"unit\":4},\"supply\":{\"magnitude\":1.0,\"unit\":18}},\"raw\":{\"signal\":{\"magnitude\":30.299736541,\"unit\":22},\"bridgeResistance\":{\"magnitude\":3689.0769444,\"unit\":28}},\"compensated\":{\"mathematicalModels\":{\"MM0123\":{\"pressure\":{\"output\":{\"magnitude\":0.109963,\"unit\":3},\"error\":{\"magnitude\":-0.0091372216,\"unit\":7}},\"temperature\":{\"output\":{\"magnitude\":39.7197,\"unit\":4},\"error\":{\"magnitude\":-0.0087145955,\"unit\":4}}}}}},{\"reference\":\"F_12300_XX_0000098765\",\"environmentTarget\":{\"pressure\":{\"magnitude\":0.19,\"unit\":3},\"temperature\":{\"magnitude\":40.0,\"unit\":4}},\"environment\":{\"pressure\":{\"magnitude\":0.190004,\"unit\":3},\"temperature\":{\"magnitude\":39.7284,\"unit\":4},\"supply\":{\"magnitude\":1.0,\"unit\":18}},\"raw\":{\"signal\":{\"magnitude\":42.177555685,\"unit\":22},\"bridgeResistance\":{\"magnitude\":3684.6154146,\"unit\":28}},\"compensated\":{\"mathematicalModels\":{\"MM0123\":{\"pressure\":{\"output\":{\"magnitude\":0.190004,\"unit\":3},\"error\":{\"magnitude\":2.3318189E-05,\"unit\":7}},\"temperature\":{\"output\":{\"magnitude\":39.7145,\"unit\":4},\"error\":{\"magnitude\":-0.013875982,\"unit\":4}}}}}},{\"reference\":\"F_12300_XX_0000098765\",\"environmentTarget\":{\"pressure\":{\"magnitude\":0.27,\"unit\":3},\"temperature\":{\"magnitude\":40.0,\"unit\":4}},\"environment\":{\"pressure\":{\"magnitude\":0.269998,\"unit\":3},\"temperature\":{\"magnitude\":39.7284,\"unit\":4},\"supply\":{\"magnitude\":1.0,\"unit\":18}},\"raw\":{\"signal\":{\"magnitude\":54.013879922,\"unit\":22},\"bridgeResistance\":{\"magnitude\":3680.2587913,\"unit\":28}},\"compensated\":{\"mathematicalModels\":{\"MM0123\":{\"pressure\":{\"output\":{\"magnitude\":0.270016,\"unit\":3},\"error\":{\"magnitude\":0.0051611949,\"unit\":7}},\"temperature\":{\"output\":{\"magnitude\":39.7128,\"unit\":4},\"error\":{\"magnitude\":-0.015632767,\"unit\":4}}}}}},{\"reference\":\"F_12300_XX_0000098765\",\"environmentTarget\":{\"pressure\":{\"magnitude\":0.35,\"unit\":3},\"temperature\":{\"magnitude\":40.0,\"unit\":4}},\"environment\":{\"pressure\":{\"magnitude\":0.350002,\"unit\":3},\"temperature\":{\"magnitude\":39.7284,\"unit\":4},\"supply\":{\"magnitude\":1.0,\"unit\":18}},\"raw\":{\"signal\":{\"magnitude\":65.805074007,\"unit\":22},\"bridgeResistance\":{\"magnitude\":3675.994032,\"unit\":28}},\"compensated\":{\"mathematicalModels\":{\"MM0123\":{\"pressure\":{\"output\":{\"magnitude\":0.349974,\"unit\":3},\"error\":{\"magnitude\":-0.0078616514,\"unit\":7}},\"temperature\":{\"output\":{\"magnitude\":39.7128,\"unit\":4},\"error\":{\"magnitude\":-0.01561436,\"unit\":4}}}}}},{\"reference\":\"F_12300_XX_0000098765\",\"environmentTarget\":{\"pressure\":{\"magnitude\":0.03,\"unit\":3},\"temperature\":{\"magnitude\":60.0,\"unit\":4}},\"environment\":{\"pressure\":{\"magnitude\":0.0299999,\"unit\":3},\"temperature\":{\"magnitude\":59.8651,\"unit\":4},\"supply\":{\"magnitude\":1.0,\"unit\":18}},\"raw\":{\"signal\":{\"magnitude\":19.604034653,\"unit\":22},\"bridgeResistance\":{\"magnitude\":3896.2995143,\"unit\":28}},\"compensated\":{\"mathematicalModels\":{\"MM0123\":{\"pressure\":{\"output\":{\"magnitude\":0.0300139,\"unit\":3},\"error\":{\"magnitude\":0.0040132125,\"unit\":7}},\"temperature\":{\"output\":{\"magnitude\":59.9337,\"unit\":4},\"error\":{\"magnitude\":0.068596457,\"unit\":4}}}}}},{\"reference\":\"F_12300_XX_0000098765\",\"environmentTarget\":{\"pressure\":{\"magnitude\":0.11,\"unit\":3},\"temperature\":{\"magnitude\":60.0,\"unit\":4}},\"environment\":{\"pressure\":{\"magnitude\":0.109995,\"unit\":3},\"temperature\":{\"magnitude\":59.8651,\"unit\":4},\"supply\":{\"magnitude\":1.0,\"unit\":18}},\"raw\":{\"signal\":{\"magnitude\":31.600949028,\"unit\":22},\"bridgeResistance\":{\"magnitude\":3891.7514685,\"unit\":28}},\"compensated\":{\"mathematicalModels\":{\"MM0123\":{\"pressure\":{\"output\":{\"magnitude\":0.109965,\"unit\":3},\"error\":{\"magnitude\":-0.008619277,\"unit\":7}},\"temperature\":{\"output\":{\"magnitude\":59.9365,\"unit\":4},\"error\":{\"magnitude\":0.071398734,\"unit\":4}}}}}},{\"reference\":\"F_12300_XX_0000098765\",\"environmentTarget\":{\"pressure\":{\"magnitude\":0.19,\"unit\":3},\"temperature\":{\"magnitude\":60.0,\"unit\":4}},\"environment\":{\"pressure\":{\"magnitude\":0.190009,\"unit\":3},\"temperature\":{\"magnitude\":59.8651,\"unit\":4},\"supply\":{\"magnitude\":1.0,\"unit\":18}},\"raw\":{\"signal\":{\"magnitude\":43.579762231,\"unit\":22},\"bridgeResistance\":{\"magnitude\":3877.2639948,\"unit\":28}},\"compensated\":{\"mathematicalModels\":{\"MM0123\":{\"pressure\":{\"output\":{\"magnitude\":0.190016,\"unit\":3},\"error\":{\"magnitude\":0.0019454055,\"unit\":7}},\"temperature\":{\"output\":{\"magnitude\":59.9394,\"unit\":4},\"error\":{\"magnitude\":0.074263125,\"unit\":4}}}}}},{\"reference\":\"F_12300_XX_0000098765\",\"environmentTarget\":{\"pressure\":{\"magnitude\":0.27,\"unit\":3},\"temperature\":{\"magnitude\":60.0,\"unit\":4}},\"environment\":{\"pressure\":{\"magnitude\":0.270006,\"unit\":3},\"temperature\":{\"magnitude\":59.8651,\"unit\":4},\"supply\":{\"magnitude\":1.0,\"unit\":18}},\"raw\":{\"signal\":{\"magnitude\":55.520057917,\"unit\":22},\"bridgeResistance\":{\"magnitude\":3872.8109489,\"unit\":28}},\"compensated\":{\"mathematicalModels\":{\"MM0123\":{\"pressure\":{\"output\":{\"magnitude\":0.270032,\"unit\":3},\"error\":{\"magnitude\":0.0075675436,\"unit\":7}},\"temperature\":{\"output\":{\"magnitude\":59.9389,\"unit\":4},\"error\":{\"magnitude\":0.073763296,\"unit\":4}}}}}},{\"reference\":\"F_12300_XX_0000098765\",\"environmentTarget\":{\"pressure\":{\"magnitude\":0.35,\"unit\":3},\"temperature\":{\"magnitude\":60.0,\"unit\":4}},\"environment\":{\"pressure\":{\"magnitude\":0.349994,\"unit\":3},\"temperature\":{\"magnitude\":59.8651,\"unit\":4},\"supply\":{\"magnitude\":1.0,\"unit\":18}},\"raw\":{\"signal\":{\"magnitude\":67.418352287,\"unit\":22},\"bridgeResistance\":{\"magnitude\":3868.4767722,\"unit\":28}},\"compensated\":{\"mathematicalModels\":{\"MM0123\":{\"pressure\":{\"output\":{\"magnitude\":0.349987,\"unit\":3},\"error\":{\"magnitude\":-0.0021229316,\"unit\":7}},\"temperature\":{\"output\":{\"magnitude\":59.9434,\"unit\":4},\"error\":{\"magnitude\":0.078304539,\"unit\":4}}}}}},{\"reference\":\"F_12300_XX_0000098765\",\"environmentTarget\":{\"pressure\":{\"magnitude\":0.03,\"unit\":3},\"temperature\":{\"magnitude\":80.0,\"unit\":4}},\"environment\":{\"pressure\":{\"magnitude\":0.0299987,\"unit\":3},\"temperature\":{\"magnitude\":79.9513,\"unit\":4},\"supply\":{\"magnitude\":1.0,\"unit\":18}},\"raw\":{\"signal\":{\"magnitude\":20.96693822,\"unit\":22},\"bridgeResistance\":{\"magnitude\":4094.2798686,\"unit\":28}},\"compensated\":{\"mathematicalModels\":{\"MM0123\":{\"pressure\":{\"output\":{\"magnitude\":0.0300202,\"unit\":3},\"error\":{\"magnitude\":0.0061545516,\"unit\":7}},\"temperature\":{\"output\":{\"magnitude\":80.0538,\"unit\":4},\"error\":{\"magnitude\":0.10242499,\"unit\":4}}}}}},{\"reference\":\"F_12300_XX_0000098765\",\"environmentTarget\":{\"pressure\":{\"magnitude\":0.11,\"unit\":3},\"temperature\":{\"magnitude\":80.0,\"unit\":4}},\"environment\":{\"pressure\":{\"magnitude\":0.110013,\"unit\":3},\"temperature\":{\"magnitude\":79.9513,\"unit\":4},\"supply\":{\"magnitude\":1.0,\"unit\":18}},\"raw\":{\"signal\":{\"magnitude\":33.086392769,\"unit\":22},\"bridgeResistance\":{\"magnitude\":4089.6557362,\"unit\":28}},\"compensated\":{\"mathematicalModels\":{\"MM0123\":{\"pressure\":{\"output\":{\"magnitude\":0.109965,\"unit\":3},\"error\":{\"magnitude\":-0.013726951,\"unit\":7}},\"temperature\":{\"output\":{\"magnitude\":80.0564,\"unit\":4},\"error\":{\"magnitude\":0.10502604,\"unit\":4}}}}}},{\"reference\":\"F_12300_XX_0000098765\",\"environmentTarget\":{\"pressure\":{\"magnitude\":0.19,\"unit\":3},\"temperature\":{\"magnitude\":80.0,\"unit\":4}},\"environment\":{\"pressure\":{\"magnitude\":0.190002,\"unit\":3},\"temperature\":{\"magnitude\":79.9513,\"unit\":4},\"supply\":{\"magnitude\":1.0,\"unit\":18}},\"raw\":{\"signal\":{\"magnitude\":45.192919898,\"unit\":22},\"bridgeResistance\":{\"magnitude\":4085.123909,\"unit\":28}},\"compensated\":{\"mathematicalModels\":{\"MM0123\":{\"pressure\":{\"output\":{\"magnitude\":0.190006,\"unit\":3},\"error\":{\"magnitude\":0.0010687773,\"unit\":7}},\"temperature\":{\"output\":{\"magnitude\":80.0643,\"unit\":4},\"error\":{\"magnitude\":0.11293662,\"unit\":4}}}}}},{\"reference\":\"F_12300_XX_0000098765\",\"environmentTarget\":{\"pressure\":{\"magnitude\":0.27,\"unit\":3},\"temperature\":{\"magnitude\":80.0,\"unit\":4}},\"environment\":{\"pressure\":{\"magnitude\":0.270003,\"unit\":3},\"temperature\":{\"magnitude\":79.9513,\"unit\":4},\"supply\":{\"magnitude\":1.0,\"unit\":18}},\"raw\":{\"signal\":{\"magnitude\":57.271028109,\"unit\":22},\"bridgeResistance\":{\"magnitude\":4080.6383175,\"unit\":28}},\"compensated\":{\"mathematicalModels\":{\"MM0123\":{\"pressure\":{\"output\":{\"magnitude\":0.270045,\"unit\":3},\"error\":{\"magnitude\":0.011980425,\"unit\":7}},\"temperature\":{\"output\":{\"magnitude\":80.0724,\"unit\":4},\"error\":{\"magnitude\":0.12109066,\"unit\":4}}}}}},{\"reference\":\"F_12300_XX_0000098765\",\"environmentTarget\":{\"pressure\":{\"magnitude\":0.35,\"unit\":3},\"temperature\":{\"magnitude\":80.0,\"unit\":4}},\"environment\":{\"pressure\":{\"magnitude\":0.350001,\"unit\":3},\"temperature\":{\"magnitude\":79.9513,\"unit\":4},\"supply\":{\"magnitude\":1.0,\"unit\":18}},\"raw\":{\"signal\":{\"magnitude\":69.304666615,\"unit\":22},\"bridgeResistance\":{\"magnitude\":4076.1600415,\"unit\":28}},\"compensated\":{\"mathematicalModels\":{\"MM0123\":{\"pressure\":{\"output\":{\"magnitude\":0.34998,\"unit\":3},\"error\":{\"magnitude\":-0.0058591743,\"unit\":7}},\"temperature\":{\"output\":{\"magnitude\":80.0765,\"unit\":4},\"error\":{\"magnitude\":0.12510468,\"unit\":4}}}}}}]},{\"version\":\"1.0.0\",\"header\":{\"creationDate\":\"2022-06-03T00:00:00\",\"remarks\":\"\",\"serialNumber\":\"98143\",\"productNumber\":\"123021.1804\",\"productType\":\"PAA-9L\",\"pressureType\":2,\"productSeries\":\"9L\",\"compensatedTemperatureRange\":{\"min\":-10.0,\"max\":80.0,\"unit\":4},\"compensatedPressureRange\":{\"min\":0.0,\"max\":0.35,\"unit\":3},\"electricSupply\":{\"magnitude\":1.0,\"unit\":18},\"orderNumber\":9990266,\"orderPosition\":3,\"orderTargetDispatchDate\":\"2022-06-02T00:00:00+00:00\",\"customerName\":\"DemoData Inc.\",\"customerNumber\":12345678,\"customerOrderNumber\":\"Cust-9990266-123\",\"customerReferenceNumber\":\"\",\"customerProductType\":\"123021-1804 Rev.AA\"},\"compensationMethods\":{\"mathematicalModels\":{\"MM0123\":{\"modelType\":\"MM0123\",\"productNumber\":\"000000.0000\",\"compensatedTemperatureRange\":{\"min\":-10.0,\"max\":80.0,\"unit\":4},\"compensatedPressureRange\":{\"min\":0.0,\"max\":0.35,\"unit\":3},\"electricSupply\":{\"magnitude\":1.0,\"unit\":18},\"parts\":{\"pressure\":{\"inputs\":[\"Sig\",\"R\"],\"output\":\"P\",\"description\":\"P = f(Sig,R)\",\"coefficients\":[[5.01094415751,-0.00515407445566,1.97589625924E-06,-3.3903578985E-10,2.18202092029E-14],[-0.180607590932,0.000194815375759,-7.55598375928E-08,1.30260258371E-11,-8.43476865996E-16],[0.000347365210426,-3.52322510315E-07,1.34928332747E-10,-2.30145933714E-14,1.47117896518E-18]]},\"temperature\":{\"inputs\":[\"R\",\"Sig\"],\"output\":\"T\",\"description\":\"T = f(R,Sig)\",\"coefficients\":[[-8355.62780258,13.1948479849,-0.151328425562],[8.23648441639,-0.0132289162835,0.000163015868308],[-0.00311044840995,4.99737890629E-06,-6.58344063029E-08],[5.31630899336E-07,-8.39693337153E-10,1.18081258333E-11],[-3.42761493955E-11,5.28910437915E-14,-7.93439241106E-16]]}}}}},\"measurements\":[{\"reference\":\"F_12300_XX_0000098765\",\"environmentTarget\":{\"pressure\":{\"magnitude\":0.03,\"unit\":3},\"temperature\":{\"magnitude\":-10.0,\"unit\":4}},\"environment\":{\"pressure\":{\"magnitude\":0.0299944,\"unit\":3},\"temperature\":{\"magnitude\":-10.7286,\"unit\":4},\"supply\":{\"magnitude\":1.0,\"unit\":18}},\"raw\":{\"signal\":{\"magnitude\":13.928380316,\"unit\":22},\"bridgeResistance\":{\"magnitude\":3273.6951896,\"unit\":28}},\"compensated\":{\"mathematicalModels\":{\"MM0123\":{\"pressure\":{\"output\":{\"magnitude\":0.0300044,\"unit\":3},\"error\":{\"magnitude\":0.0028578761,\"unit\":7}},\"temperature\":{\"output\":{\"magnitude\":-10.8297,\"
